vi "Lighting Enable.vi"(7 "Enabled?":bool, 8 "error in (no error)":errorcluster, 10 "Enable light Refnum":refnum<vi>, 11 "Light List Refnum":refnum<vi>) -> (0 "error out":errorcluster)   [LabVIEW 2020, in "3D Plot.lvclass"]
uses:
  3D Plot.lvclass
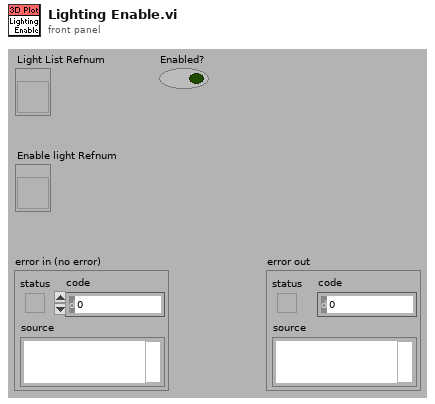
[diagram p1: front panel]
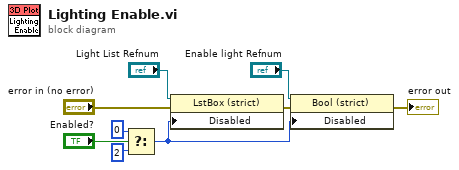
[diagram p0: block diagram]
diagram:
  n1 = Select(t=u8 0 ("Disabled"), s="Enabled?", f=u8 2) -> (s? t:f=w4:u8)
  n2 = property on="Property Node" class="LstBox (strict)"(reference="Light List Refnum", error in="error in (no error)", "Disabled"=w4) -> (error out=w7:errorcluster)  [unwired: 1 out]
  n3 = property on="Property Node" class="Bool (strict)"(reference="Enable light Refnum", error in=w7, "Disabled"=w4) -> (error out=→"error out":errorcluster)  [unwired: 1 out]
